vi "EscapeBuffer.vi"(8 "FrameByte":u8, 9 "XORByte":u8, 10 "EscapeByte":u8, 11 "In":u8[](array[numeric])) -> (3 "Out":u8[](array[numeric]))   [LabVIEW 2009]
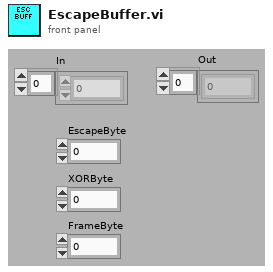
[diagram p1: front panel]
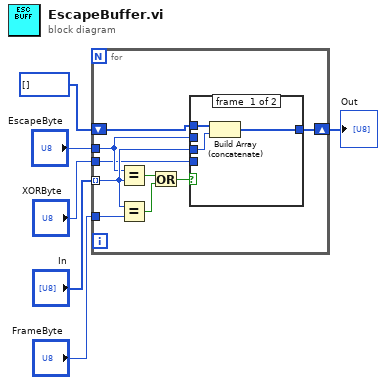
[diagram p0: block diagram]
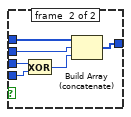
[diagram p2: hidden frame]
diagram:
  n1 = for {
    tunnel: "In" -> [w10] mode=indexing
    tunnel: "EscapeByte" -> [w8]
    tunnel: "FrameByte" -> [w15]
    shift-right: [w9] -> w2
    shift-left: u8[] [] ("Out") -> [w11]
    tunnel: "XORByte" -> [w7]
    n2 = Equal?(x=w8, y=w10) -> (x = y?=w14:bool)
    n3 = Equal?(x=w10, y=w15) -> (x = y?=w13:bool)
    n4 = Or(x=w14, y=w13) -> (x .or. y?=w12:bool)
    n5 = case shown="True" w12 {
      tunnel: w11 -> [w18 w24]
      tunnel: w10 -> [w17 w21]
      tunnel: [w16 w23] -> w9
      tunnel: w8 -> [_ w22]
      tunnel: w7 -> [_ w20]
      frame #0 {
        n6 = Build Array (concatenate)(w18, w17) -> (w16:u8[])
      }
      frame #1 {
        n7 = Exclusive Or(1:w20, 2:w21) -> (0:w19:u8)
        n8 = Build Array (concatenate)(w24, w22, w19) -> (w23:u8[])
      }
    }
  }
  "Out" <- w2
